vi "Drive.vi"(8 "error in":errorcluster, 10 "Sensors":T1={"Gyro"={"DevStatus"={"status"=FALSE, "code"=0, "source"=""}, "Analog Module"=enum."Controller 1", "Analog Channel"=enum."Invalid", "Offset"=0.0, "Gain (VoltsPerDegree/Second)"=0.0}, "Encoders"={"Left Drive CAN"={"DeviceStatus"={"status"=FALSE, "code"=0, "source"=""}, "Type"=enum."PWM", "PWM"={"Controller"=enum."Controller 1", "PWM Channel"=enum."PWM 1", "DeadBand"={"Name"="", "maxPositivePwm"=0, "minPositivePwm"=0, "centerPwm"=0, "maxNegativePwm"=0, "minNegativePwm"=0, "angularRange"=0}}, "CAN"={"Device Number"=0, "Control Mode"=enum."Percent VBus", "Semaphore"=refnum, "Max Vout"=12.0, "TalonSRX Control Mode"=enum."Percent VBus"}, "Invert"=FALSE, "TransformRef"=refnum, "InvTransformRef"=refnum}, "Right Drive CAN"={"DeviceStatus"={"status"=FALSE, "code"=0, "source"=""}, "Type"=enum."PWM", "PWM"={"Controller"=enum."Controller 1", "PWM Channel"=enum."PWM 1", "DeadBand"={"Name"="", "maxPositivePwm"=0, "minPositivePwm"=0, "centerPwm"=0, "maxNegativePwm"=0, "minNegativePwm"=0, "angularRange"=0}}, "CAN"={"Device Number"=0, "Control Mode"=enum."Percent VBus", "Semaphore"=refnum, "Max Vout"=12.0, "TalonSRX Control Mode"=enum."Percent VBus"}, "Invert"=FALSE, "TransformRef"=refnum, "InvTransformRef"=refnum}, "Strafe CAN"={"DeviceStatus"={"status"=FALSE, "code"=0, "source"=""}, "Type"=enum."PWM", "PWM"={"Controller"=enum."Controller 1", "PWM Channel"=enum."PWM 1", "DeadBand"={"Name"="", "maxPositivePwm"=0, "minPositivePwm"=0, "centerPwm"=0, "maxNegativePwm"=0, "minNegativePwm"=0, "angularRange"=0}}, "CAN"={"Device Number"=0, "Control Mode"=enum."Percent VBus", "Semaphore"=refnum, "Max Vout"=12.0, "TalonSRX Control Mode"=enum."Percent VBus"}, "Invert"=FALSE, "TransformRef"=refnum, "InvTransformRef"=refnum}, "Elevator CAN"={"DeviceStatus"={"status"=FALSE, "code"=0, "source"=""}, "Type"=enum."PWM", "PWM"={"Controller"=enum."Controller 1", "PWM Channel"=enum."PWM 1", "DeadBand"={"Name"="", "maxPositivePwm"=0, "minPositivePwm"=0, "centerPwm"=0, "maxNegativePwm"=0, "minNegativePwm"=0, "angularRange"=0}}, "CAN"={"Device Number"=0, "Control Mode"=enum."Percent VBus", "Semaphore"=refnum, "Max Vout"=12.0, "TalonSRX Control Mode"=enum."Percent VBus"}, "Invert"=FALSE, "TransformRef"=refnum, "InvTransformRef"=refnum}}, "Switches"={"Elevator Top"={"DevStatus"={"status"=FALSE, "code"=0, "source"=""}, "DIO Channel"=enum."DIO 1", "Controller"=enum."Controller 1", "CntIndex"=enum."Invalid", "Normally Closed"=FALSE}, "Elevator Bottom"={"DevStatus"={"status"=FALSE, "code"=0, "source"=""}, "DIO Channel"=enum."DIO 1", "Controller"=enum."Controller 1", "CntIndex"=enum."Invalid", "Normally Closed"=FALSE}, "Claw Outside"={"DevStatus"={"status"=FALSE, "code"=0, "source"=""}, "DIO Channel"=enum."DIO 1", "Controller"=enum."Controller 1", "CntIndex"=enum."Invalid", "Normally Closed"=FALSE}}, "Arm Capper Pot"={"DevStatus"={"status"=FALSE, "code"=0, "source"=""}, "Controller"=enum."Controller 1", "Analog Channel"=enum."Invalid", "Invert Output"=FALSE}, "Arm Angle Pot"={"DevStatus"={"status"=FALSE, "code"=0, "source"=""}, "Controller"=enum."Controller 1", "Analog Channel"=enum."Invalid", "Invert Output"=FALSE}, "Sonar"={"Front"={"AIDeviceRef"={"DevStatus"={"status"=FALSE, "code"=0, "source"=""}, "Controller"=enum."Controller 1", "Analog Channel"=enum."Invalid"}, "Scaling factor (V/in)"=0.0098, "Average Bits"=3}, "Back"={"AIDeviceRef"={"DevStatus"={"status"=FALSE, "code"=0, "source"=""}, "Controller"=enum."Controller 1", "Analog Channel"=enum."Invalid"}, "Scaling factor (V/in)"=0.0098, "Average Bits"=3}}} {"Sonar"."Back"."Average Bits" max=15; "Sonar"."Front"."Average Bits" max=15}, 11 "Actuators":T20={"Drive"={"DevStatus"={"status"=FALSE, "code"=0, "source"=""}, "Motors[]"=[], "Square Inputs"=FALSE, "Max Output"=1.0}, "Strafe"={"DeviceStatus"={"status"=FALSE, "code"=0, "source"=""}, "Type"=enum."PWM", "PWM"={"Controller"=enum."Controller 1", "PWM Channel"=enum."Invalid", "DeadBand"={"Name"="", "maxPositivePwm"=0, "minPositivePwm"=0, "centerPwm"=0, "maxNegativePwm"=0, "minNegativePwm"=0, "angularRange"=0}}, "CAN"={"Device Number"=0, "Control Mode"=enum."Percent VBus", "Semaphore"=refnum, "Max Vout"=12.0, "TalonSRX Control Mode"=enum."Percent VBus"}, "Invert"=FALSE, "TransformRef"=refnum, "InvTransformRef"=refnum}, "Elevator Left"={"DeviceStatus"={"status"=FALSE, "code"=0, "source"=""}, "Type"=enum."PWM", "PWM"={"Controller"=enum."Controller 1", "PWM Channel"=enum."Invalid", "DeadBand"={"Name"="", "maxPositivePwm"=0, "minPositivePwm"=0, "centerPwm"=0, "maxNegativePwm"=0, "minNegativePwm"=0, "angularRange"=0}}, "CAN"={"Device Number"=0, "Control Mode"=enum."Percent VBus", "Semaphore"=refnum, "Max Vout"=12.0, "TalonSRX Control Mode"=enum."Percent VBus"}, "Invert"=FALSE, "TransformRef"=refnum, "InvTransformRef"=refnum}, "Elevator Right"={"DeviceStatus"={"status"=FALSE, "code"=0, "source"=""}, "Type"=enum."PWM", "PWM"={"Controller"=enum."Controller 1", "PWM Channel"=enum."Invalid", "DeadBand"={"Name"="", "maxPositivePwm"=0, "minPositivePwm"=0, "centerPwm"=0, "maxNegativePwm"=0, "minNegativePwm"=0, "angularRange"=0}}, "CAN"={"Device Number"=0, "Control Mode"=enum."Percent VBus", "Semaphore"=refnum, "Max Vout"=12.0, "TalonSRX Control Mode"=enum."Percent VBus"}, "Invert"=FALSE, "TransformRef"=refnum, "InvTransformRef"=refnum}, "Arm Clapper"={"DeviceStatus"={"status"=FALSE, "code"=0, "source"=""}, "Type"=enum."PWM", "PWM"={"Controller"=enum."Controller 1", "PWM Channel"=enum."Invalid", "DeadBand"={"Name"="", "maxPositivePwm"=0, "minPositivePwm"=0, "centerPwm"=0, "maxNegativePwm"=0, "minNegativePwm"=0, "angularRange"=0}}, "CAN"={"Device Number"=0, "Control Mode"=enum."Percent VBus", "Semaphore"=refnum, "Max Vout"=12.0, "TalonSRX Control Mode"=enum."Percent VBus"}, "Invert"=FALSE, "TransformRef"=refnum, "InvTransformRef"=refnum}, "Arm Angle"={"DeviceStatus"={"status"=FALSE, "code"=0, "source"=""}, "Type"=enum."PWM", "PWM"={"Controller"=enum."Controller 1", "PWM Channel"=enum."Invalid", "DeadBand"={"Name"="", "maxPositivePwm"=0, "minPositivePwm"=0, "centerPwm"=0, "maxNegativePwm"=0, "minNegativePwm"=0, "angularRange"=0}}, "CAN"={"Device Number"=0, "Control Mode"=enum."Percent VBus", "Semaphore"=refnum, "Max Vout"=12.0, "TalonSRX Control Mode"=enum."Percent VBus"}, "Invert"=FALSE, "TransformRef"=refnum, "InvTransformRef"=refnum}, "Arm Roller Left"={"DeviceStatus"={"status"=FALSE, "code"=0, "source"=""}, "Type"=enum."PWM", "PWM"={"Controller"=enum."Controller 1", "PWM Channel"=enum."Invalid", "DeadBand"={"Name"="", "maxPositivePwm"=0, "minPositivePwm"=0, "centerPwm"=0, "maxNegativePwm"=0, "minNegativePwm"=0, "angularRange"=0}}, "CAN"={"Device Number"=0, "Control Mode"=enum."Percent VBus", "Semaphore"=refnum, "Max Vout"=12.0, "TalonSRX Control Mode"=enum."Percent VBus"}, "Invert"=FALSE, "TransformRef"=refnum, "InvTransformRef"=refnum}, "Arm Roller Right"={"DeviceStatus"={"status"=FALSE, "code"=0, "source"=""}, "Type"=enum."PWM", "PWM"={"Controller"=enum."Controller 1", "PWM Channel"=enum."Invalid", "DeadBand"={"Name"="", "maxPositivePwm"=0, "minPositivePwm"=0, "centerPwm"=0, "maxNegativePwm"=0, "minNegativePwm"=0, "angularRange"=0}}, "CAN"={"Device Number"=0, "Control Mode"=enum."Percent VBus", "Semaphore"=refnum, "Max Vout"=12.0, "TalonSRX Control Mode"=enum."Percent VBus"}, "Invert"=FALSE, "TransformRef"=refnum, "InvTransformRef"=refnum}}) -> ()   [LabVIEW 2014]
doc: "Drivetrain and strafe control loop.\nGathers joystick and gyro inputs and controls the left / right drive and strafe motors."
uses:
  Utilities/Actuators.ctl
  <vilib>/Rock Robotics/WPI/RobotDrive/WPI_RobotDriveDevRef.ctl
  <vilib>/Rock Robotics/WPI/MotorControl/WPI_MotorControlDeviceRef.ctl
  <vilib>/Rock Robotics/WPI/MotorControl/WPI_MotorControlType.ctl
  <vilib>/Rock Robotics/SystemInterfaces/Typedef/FPGA_TypedefDigitalModule.ctl
  <vilib>/Rock Robotics/SystemInterfaces/DIO/FPGA_DIOPWMChannel.ctl
  <vilib>/Rock Robotics/WPI/PWM/WPI_PWMDeadband.ctl
  <vilib>/Rock Robotics/WPI/CAN/Jaguar/SubVIs/WPI_CANJaguar_ControlMode.ctl
  <vilib>/Rock Robotics/WPI/CAN/TalonSRX/WPI_CANTalonSRX_APIControlMode.ctl
  <vilib>/Rock Robotics/WPI/PWM/WPI_PWMTransform_ConPane.ctl
  Utilities/Sensors.ctl
  <vilib>/Rock Robotics/WPI/Gyro/WPI_GyroDevRef.ctl
  <vilib>/Rock Robotics/SystemInterfaces/Typedef/FPGA_TypedefAnalogModule.ctl
  <vilib>/Rock Robotics/SystemInterfaces/AI/FPGA_AIChannel.ctl
  <vilib>/Rock Robotics/WPI/Switch/WPI_SwitchDevRef.ctl
  <vilib>/Rock Robotics/SystemInterfaces/DIO/FPGA_DIOChannel.ctl
  <vilib>/Rock Robotics/SystemInterfaces/Counter/FPGA_CounterCtrSystemIndex.ctl
  <vilib>/Rock Robotics/WPI/Potentiometer/WPI_PotentiometerDevRef.ctl
  <vilib>/Rock Robotics/WPI/Ultrasonic/WPI_SonarMB1010AnalogDeviceRef.ctl
  <vilib>/Rock Robotics/WPI/AnalogChannel/WPI_AnalogChannelDevRef.ctl
  Drive Output Data.ctl
  Robot Global Data.vi
panel:
  in  "Proportional":dbl=1.0 format="%#_13g"
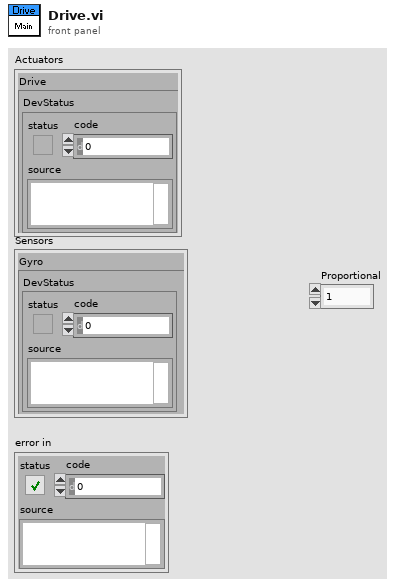
[diagram p1: front panel]
types:
  T1 = typedef "Sensors.ctl" = cluster{"Gyro":T2, "Encoders":cluster{"Left Drive CAN":T5, "Right Drive CAN":T5, "Strafe CAN":T5, "Elevator CAN":T5}, "Switches":cluster{"Elevator Top":T14, "Elevator Bottom":T14, "Claw Outside":T14}, "Arm Capper Pot":T17, "Arm Angle Pot":T17, "Sonar":cluster{"Front":T18, "Back":T18}}
  T2 = typedef "WPI_GyroDevRef.ctl" = cluster{"DevStatus":errorcluster, "Analog Module":T3, "Analog Channel":T4, "Offset":dbl, "Gain (VoltsPerDegree/Second)":dbl}
  T3 = typedef "FPGA_TypedefAnalogModule.ctl" = enum16{"Controller 1"}
  T4 = typedef "FPGA_AIChannel.ctl" = enum8{"AI 0", "AI 1", "AI 2", "AI 3", "AI MXP 0", "AI MXP 1", "AI MXP 2", "AI MXP 3", "Invalid"}
  T5 = typedef "WPI_MotorControlDeviceRef.ctl" = cluster{"DeviceStatus":errorcluster, "Type":T6, "PWM":cluster{"Controller":T7, "PWM Channel":T8, "DeadBand":T9}, "CAN":cluster{"Device Number":u8, "Control Mode":T10, "Semaphore":T11, "Max Vout":dbl, "TalonSRX Control Mode":T12}, "Invert":bool, "TransformRef":T13, "InvTransformRef":T13}
  T6 = typedef "WPI_MotorControlType.ctl" = enum16{"PWM", "CAN", "CANTalonSRX"}
  T7 = typedef "FPGA_TypedefDigitalModule.ctl" = enum16{"Controller 1"}
  T8 = typedef "FPGA_DIOPWMChannel.ctl" = enum8{"PWM 0", "PWM 1", "PWM 2", "PWM 3", "PWM 4", "PWM 5", "PWM 6", "PWM 7", "PWM 8", "PWM 9", "PWM MXP 0", "PWM MXP 1", "PWM MXP 2", "PWM MXP 3", "PWM MXP 4", "PWM MXP 5", "PWM MXP 6", "PWM MXP 7", "PWM MXP 8", "PWM MXP 9", "Invalid"}
  T9 = typedef "WPI_PWMDeadband.ctl" = cluster{"Name":string, "maxPositivePwm":i32, "minPositivePwm":i32, "centerPwm":i32, "maxNegativePwm":i32, "minNegativePwm":i32, "angularRange":u16}
  T10 = typedef "WPI_CANJaguar_ControlMode.ctl" = enum8{"Percent VBus", "Current", "Speed", "Position", "Voltage"}
  T11 = typedef "Semaphore RefNum" = refnum<k1>
  T12 = typedef "WPI_CANTalonSRX_APIControlMode.ctl" = enum8{"Percent VBus", "Speed", "Position", "Slave", "Unchanged / Invalid"}
  T13 = typedef "WPI_PWMTransform_ConPane.ctl" = refnum<vi>
  T14 = typedef "WPI_SwitchDevRef.ctl" = cluster{"DevStatus":errorcluster, "DIO Channel":T15, "Controller":T7, "CntIndex":T16, "Normally Closed":bool}
  T15 = typedef "FPGA_DIOChannel.ctl" = enum8{"DIO 0", "DIO 1", "DIO 2", "DIO 3", "DIO 4", "DIO 5", "DIO 6", "DIO 7", "DIO 8", "DIO 9", "DIO MXP 0", "DIO MXP 1", "DIO MXP 2", "DIO MXP 3", "DIO MXP 4", "DIO MXP 5", "DIO MXP 6", "DIO MXP 7", "DIO MXP 8", "DIO MXP 9", "DIO MXP 10", "DIO MXP 11", "DIO MXP 12", "DIO MXP 13", "DIO MXP 14", "DIO MXP 15", "Invalid"}
  T16 = typedef "FPGA_CounterCtrSystemIndex.ctl" = enum8{"Ctr 0", "Ctr 1", "Ctr 2", "Ctr 3", "Ctr 4", "Ctr 5", "Ctr 6", "Ctr 7", "Invalid"}
  T17 = typedef "WPI_PotentiometerDevRef.ctl" = cluster{"DevStatus":errorcluster, "Controller":T3, "Analog Channel":T4, "Invert Output":bool}
  T18 = typedef "WPI_SonarMB1010AnalogDeviceRef.ctl" = cluster{"AIDeviceRef":T19, "Scaling factor (V/in)":dbl, "Average Bits":u8}
  T19 = typedef "WPI_AnalogChannelDevRef.ctl" = cluster{"DevStatus":errorcluster, "Controller":T3, "Analog Channel":T4}
  T20 = typedef "Actuators.ctl" = cluster{"Drive":T21, "Strafe":T5, "Elevator Left":T5, "Elevator Right":T5, "Arm Clapper":T5, "Arm Angle":T5, "Arm Roller Left":T5, "Arm Roller Right":T5}
  T21 = typedef "WPI_RobotDriveDevRef.ctl" = cluster{"DevStatus":errorcluster, "Motors[]":T5[], "Square Inputs":bool, "Max Output":dbl}
  T22 = typedef "Drive Output Data.ctl" = cluster{"Throttle":dbl, "Rotation":dbl, "Strafe":dbl}
  T23 = typedef "WPI_DriverStationRobotMode2.ctl" = enum16{"Autonomous Disabled", "Autonomous Enabled", "Teleop Disabled", "Teleop Enabled", "Disconnected", "Finish", "Test Disabled", "Test Enabled", "Emergency Stopped"}
  T24 = typedef "Drive Input Data.ctl" = cluster{"Right Joystick X":dbl, "Left Joystick X":dbl, "Left Joystick Y":dbl, "Gyro Angle":dbl, "Half Drive":bool, "Motor Ramp?":bool}
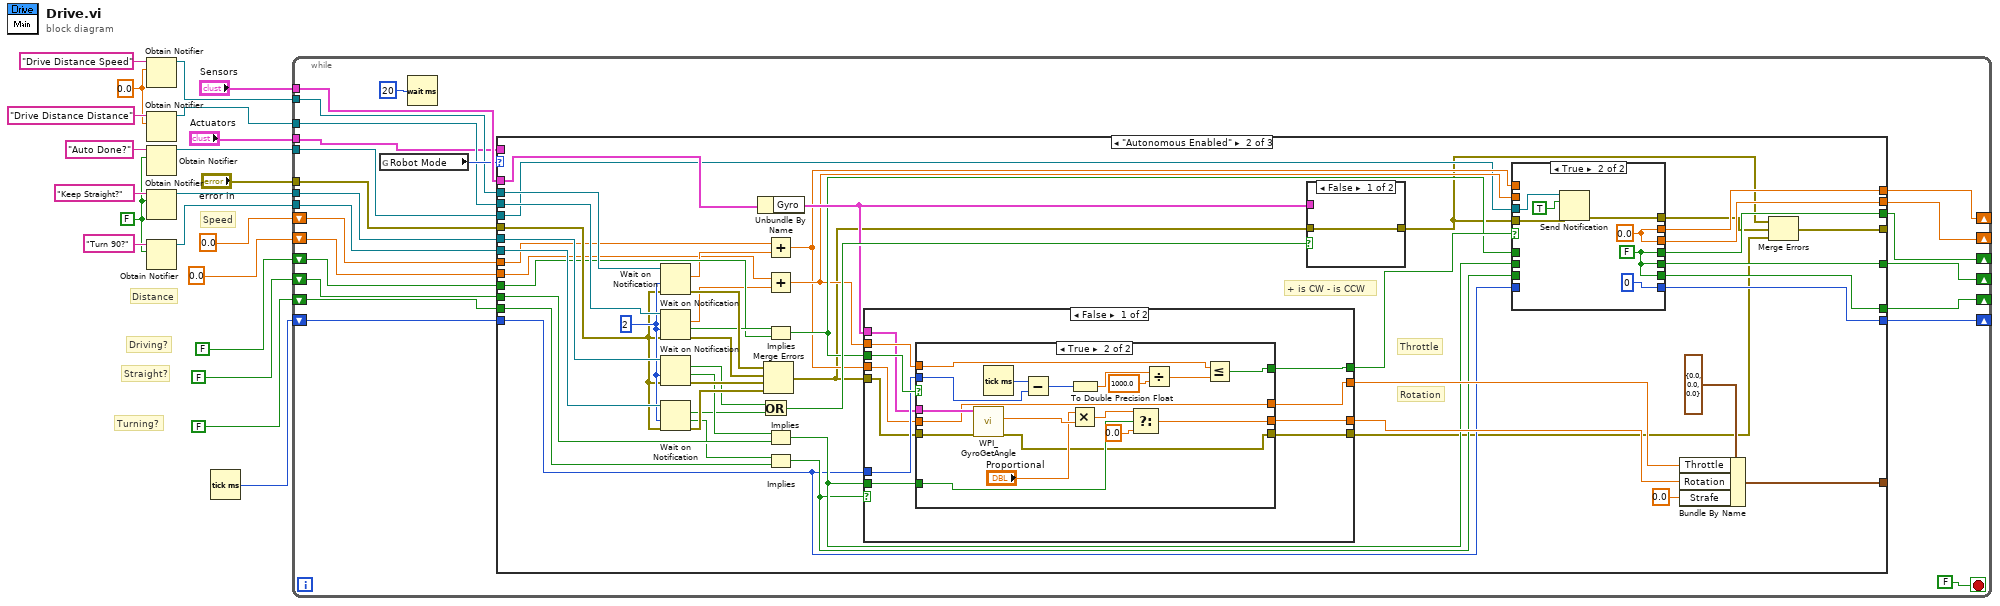
[diagram p0: block diagram]
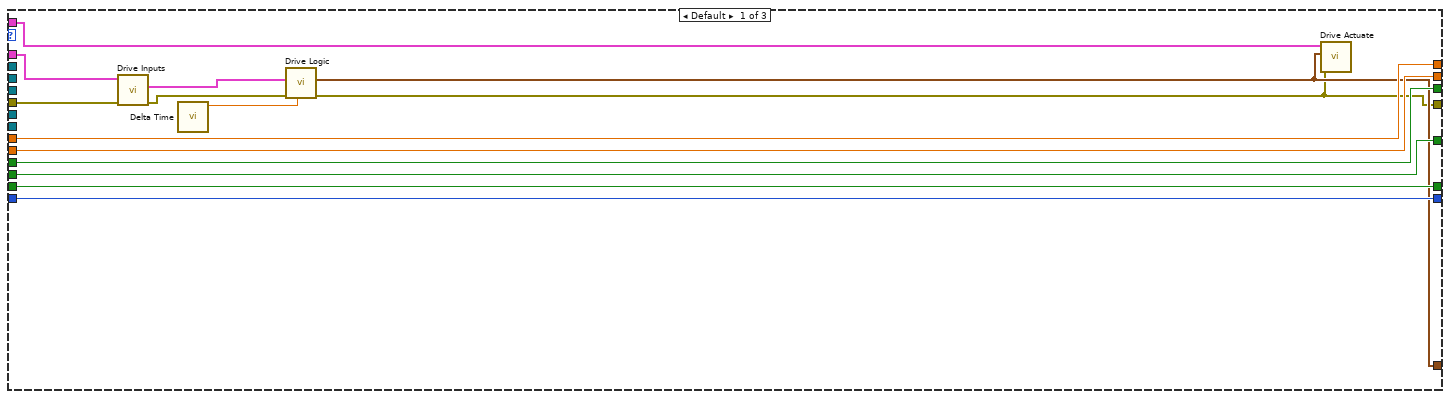
[diagram p2: hidden frame]
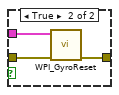
[diagram p4: hidden frame]
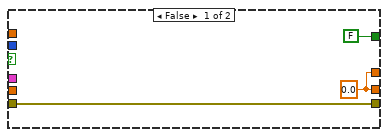
[diagram p5: hidden frame]
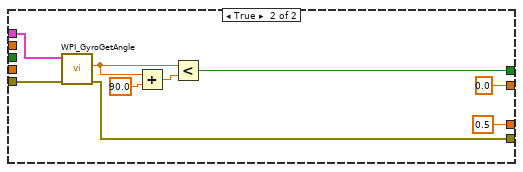
[diagram p6: hidden frame]
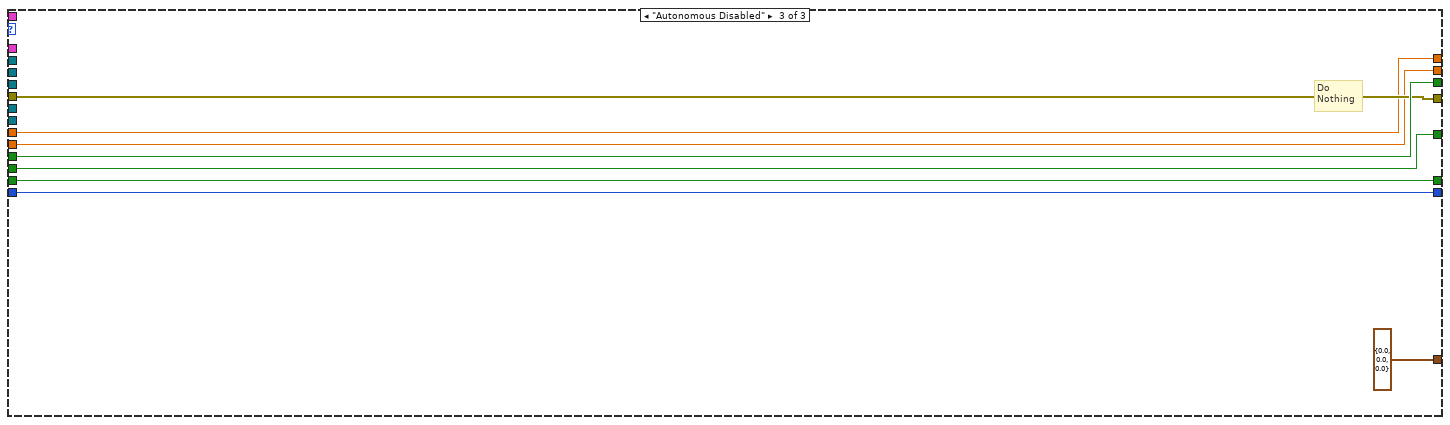
[diagram p7: hidden frame]
diagram:
  w12 = FALSE
  w13 = 0.0
  # "Speed"
  # "Distance"
  # "Driving?"
  # "Straight?"
  # "Turning?"
  n1 = Obtain Notifier(name (unnamed)="Drive Distance Speed", notification data type=w13) -> (notifier out=w11:refnum<notifier>)  [unwired: 2 in, 2 out]
  n2 = Obtain Notifier(name (unnamed)="Drive Distance Distance", notification data type=w13) -> (notifier out=w10:refnum<notifier>)  [unwired: 2 in, 2 out]
  n3 = Obtain Notifier(name (unnamed)="Auto Done?", notification data type=w12) -> (notifier out=w1:refnum<notifier>)  [unwired: 2 in, 2 out]
  n4 = Obtain Notifier(name (unnamed)="Keep Straight?", notification data type=w12) -> (notifier out=w9:refnum<notifier>)  [unwired: 2 in, 2 out]
  n5 = Obtain Notifier(name (unnamed)="Turn 90?", notification data type=w12) -> (notifier out=w8:refnum<notifier>)  [unwired: 2 in, 2 out]
  n6 = Tick Count (ms)() -> (millisecond timer value=w2:u32)
  n7 = while {
    tunnel: "error in" -> [w42]
    tunnel: "Actuators" -> [w22]
    tunnel: "Sensors" -> [w43]
    tunnel: w11 -> [w39]
    tunnel: w10 -> [w38]
    tunnel: w9 -> [w37]
    tunnel: w8 -> [w36]
    shift-right: [w34] -> _
    shift-left: FALSE -> [w35]
    shift-right: [w32] -> _
    shift-left: FALSE -> [w33]
    shift-right: [w30] -> _
    shift-left: FALSE -> [w31]
    shift-right: [w29] -> _
    shift-left: 0.0 -> [w27]
    shift-right: [w28] -> _
    shift-left: 0.0 -> [w26]
    shift-right: [w24] -> _
    shift-left: w2 -> [w25]
    tunnel: w1 -> [w23]
    stop <- FALSE stop-if-true
    n8 = global read "Robot Global Data.vi" "Robot Mode"() -> (w40:T23)
    n9 = Wait (ms)(milliseconds to wait=u32 20) -> ()  [unwired: 1 out]
    n10 = case shown="\"Autonomous Enabled\"" w40 {
      tunnel: w43 -> [w56 w102 _]
      tunnel: w42 -> [w55 w101 w171]
      tunnel: w39 -> [_ w107 _]
      tunnel: w38 -> [_ w106 _]
      tunnel: w37 -> [_ w105 _]
      tunnel: w36 -> [_ w104 _]
      tunnel: w35 -> [w53 w93 w174]
      tunnel: [w53 w74 w174] -> w34
      tunnel: w33 -> [w52 w95 w173]
      tunnel: [w52 w75 w173] -> w32
      tunnel: w31 -> [w51 w91 w172]
      tunnel: [w51 w76 w172] -> w30
      tunnel: [w50 w65 w169] -> w29
      tunnel: [w49 w67 w170] -> w28
      tunnel: w27 -> [w50 w90 w169]
      tunnel: w26 -> [w49 w87 w170]
      tunnel: w25 -> [w48 w70 w167]
      tunnel: [w46 w63 w171] -> _
      tunnel: [w47 w81 T22 {"Throttle"=0.0, "Rotation"=0.0, "Strafe"=0.0} ("Drive Outputs")] -> _
      tunnel: [w48 w69 w167] -> w24
      tunnel: w23 -> [_ w61 _]
      tunnel: w22 -> [w45 _ _]
      frame Default {
        n11 = call "Drive Inputs.vi"("error in (no error)"=w55, "Sensors"=w56) -> ("error out"=w57:errorcluster, "Drive Inputs"=w58:T24)  [unwired: 8 in]
        n12 = call "Delta Time.vi"() -> ("dt (s)"=w54:dbl)  [unwired: 11 in]
        n13 = call "Drive Logic.vi"("dt (s)"=w54, "error in (no error)"=w57, "Drive Inputs"=w58) -> ("error out"=w46:errorcluster, "Drive Outputs"=w47:T22)  [unwired: 7 in]
        n14 = call "Drive Actuate.vi"("error in"=w46, "Drive Outputs"=w47, "Actuators"=w45) -> ()  [unwired: 8 in, 1 out]
      }
      frame "Autonomous Enabled" {
        w103 = 2
        # "+ is CW - is CCW"
        # "Rotation"
        # "Throttle"
        n15 = Wait on Notification(notifier=w107, timeout in ms (-1)=w103, error in (no error)=w101) -> (notification=w89:dbl, error out=w99:errorcluster)  [unwired: 1 in, 2 out]
        n16 = Wait on Notification(notifier=w106, timeout in ms (-1)=w103, error in (no error)=w101) -> (notification=w88:dbl, timed out?=w92:bool, error out=w100:errorcluster)  [unwired: 1 in, 1 out]
        n17 = Wait on Notification(notifier=w105, timeout in ms (-1)=w103, error in (no error)=w101) -> (notification=w86:bool, timed out?=w96:bool, error out=w98:errorcluster)  [unwired: 1 in, 1 out]
        n18 = Wait on Notification(notifier=w104, timeout in ms (-1)=w103, error in (no error)=w101) -> (notification=w85:bool, timed out?=w94:bool, error out=w97:errorcluster)  [unwired: 1 in, 1 out]
        n19 = Unbundle By Name(w102) -> ("Gyro"=w83:T2)
        n20 = Or(x=w86, y=w85) -> (x .or. y?=w84:bool)
        n21 = Merge Errors(w99, w100, w98, w97) -> (w64:errorcluster)
        n22 = Add(x=w90, y=w89) -> (x+y=w66:dbl)
        n23 = Add(x=w87, y=w88) -> (x+y=w68:dbl)
        n24 = Implies(1:w91, 2:w92) -> (0:w73:bool)
        n25 = Implies(1:w95, 2:w96) -> (0:w72:bool)
        n26 = Implies(1:w93, 2:w94) -> (0:w71:bool)
        n27 = case shown="False" w71 {
          tunnel: w83 -> [w133 w162]
          tunnel: w64 -> [w132 w163]
          tunnel: w73 -> [w136 _]
          tunnel: w70 -> [w135 _]
          tunnel: w68 -> [w134 _]
          tunnel: [w131 w161] -> w77
          tunnel: [w130 0.5 ("X axis value")] -> w79
          tunnel: w66 -> [w129 _]
          tunnel: [w128 0.0 ("Y axis value")] -> w80
          tunnel: w72 -> [w127 _]
          tunnel: [w126 w158] -> w62
          frame False {
            n28 = case shown="True" w136 {
              tunnel: w135 -> [_ w156]
              tunnel: w134 -> [_ w155]
              tunnel: w133 -> [_ w147]
              tunnel: w132 -> [w137 w150]
              tunnel: [FALSE w146] -> w131
              tunnel: [w138 w142] -> w130
              tunnel: w129 -> [_ w145]
              tunnel: [w138 w145] -> w128
              tunnel: w127 -> [_ w144]
              tunnel: [w137 w140] -> w126
              frame False {
                w138 = 0.0
              }
              frame True {
                n29 = call <vilib>:"WPI_GyroGetAngle.vi"("error in (no error)"=w150, "GyroDevRef"=w147) -> ("error out"=w140:errorcluster, "Angle"=w149:dbl)  [unwired: 6 in, 2 out]
                n30 = Tick Count (ms)() -> (millisecond timer value=w157:u32)
                n31 = Subtract(x=w157, y=w156) -> (x-y=w153:u32)
                n32 = Multiply(x="Proportional", y=w149) -> (x*y=w143:dbl)
                n33 = To Double Precision Float(number=w153) -> (double precision float=w151:dbl)
                n34 = Select(t=w143, s=w144, f=0.0) -> (s? t:f=w142:dbl)
                n35 = Divide(x=w151, y=1000.0) -> (x/y=w152:dbl)
                n36 = Less Or Equal?(x=w155, y=w152) -> (x <= y?=w146:bool)
              }
            }
          }
          frame True {
            n37 = call <vilib>:"WPI_GyroGetAngle.vi"("error in (no error)"=w163, "GyroDevRef"=w162) -> ("error out"=w158:errorcluster, "Angle"=w164:dbl)  [unwired: 6 in, 2 out]
            n38 = Add(x=w164, y=90.0) -> (x+y=w166:dbl)
            n39 = Less?(x=w164, y=w166) -> (x < y?=w161:bool)
          }
        }
        n40 = case shown="False" w84 {
          tunnel: w83 -> [_ w125]
          tunnel: w64 -> [w122 w124]
          tunnel: [w122 w123] -> w59
          frame False {
          }
          frame True {
            n41 = call <vilib>:"WPI_GyroReset.vi"("error in (no error)"=w124, "GyroDevRef"=w125) -> ("error out"=w123:errorcluster)  [unwired: 8 in, 1 out]
          }
        }
        n42 = case shown="True" w77 {
          tunnel: [w114 w121] -> w76
          tunnel: [w113 w121] -> w75
          tunnel: [w112 w121] -> w74
          tunnel: w73 -> [w114 _]
          tunnel: w72 -> [w113 _]
          tunnel: w71 -> [w112 _]
          tunnel: w70 -> [w111 _]
          tunnel: [w111 u32 0 ("millisecond timer value")] -> w69
          tunnel: w68 -> [w110 _]
          tunnel: [w110 w119] -> w67
          tunnel: w66 -> [w109 _]
          tunnel: [w109 w119] -> w65
          tunnel: w61 -> [_ w118]
          tunnel: w59 -> [w108 w117]
          tunnel: [w108 w116] -> w60
          frame False {
          }
          frame True {
            w119 = 0.0
            w121 = FALSE
            n43 = Send Notification(notification=TRUE, notifier=w118, error in (no error)=w117) -> (error out=w116:errorcluster)  [unwired: 1 out]
          }
        }
        n44 = Bundle By Name(cluster=T22 {"Throttle"=0.0, "Rotation"=0.0, "Strafe"=0.0} ("Drive Outputs"), "Throttle"=w80, "Rotation"=w79, "Strafe"=0.0) -> (w81:T22)
        n45 = Merge Errors(w59, w60, w62) -> (w63:errorcluster)
      }
      frame "Autonomous Disabled" {
        # "Do\nNothing"
      }
    }
  }
